vi "InitializeCamera.vi"(8 "error in (no error)":errorcluster, 11 "CameraSession in":refnum<class "CS250-CameraHardwareClass.lvclass">) -> (0 "error out":errorcluster, 3 "CameraSession out":refnum<class "CS250-CameraHardwareClass.lvclass">)   [LabVIEW 2013, in "CS250-CameraHardwareClass.lvclass"]
doc: "This VI initializes the communication with the camera and retreives the region size"
uses:
  CS250-CameraHardwareClass.lvclass
  SubVis/DLL Calls/PARAM_ID_TypDef.ctl
  CS250-CameraHardwareClass.lvclass/CS250-CameraHardwareClass.ctl
  SubVis/CamCluster.ctl
  <vilib>/vision/Image Controls.llb/IMAQ Image.ctl
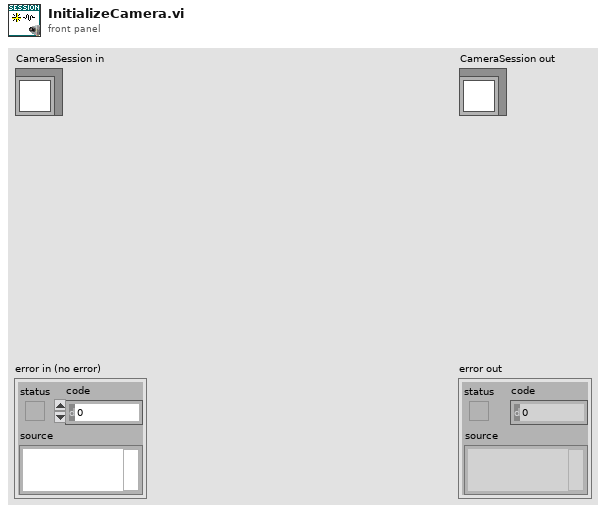
[diagram p1: front panel]
types:
  T1 = typedef "PARAM_ID_TypDef.ctl" = u32
  T2 = typedef "CamCluster.ctl" = cluster{"hcam out":i16, "TempImage":T3, "Pointer":u32, "exp_bytes out":u32, "rgn_array":cluster{"s1":u16, "s2":u16, "sbin":u16, "p1":u16, "p2":u16, "pbin":u16}, "CameraName":string}
  T3 = typedef "IMAQ Image.ctl" = refnum<image>
  T4 = cluster{"s1":u16, "s2":u16, "sbin":u16, "p1":u16, "p2":u16, "pbin":u16}
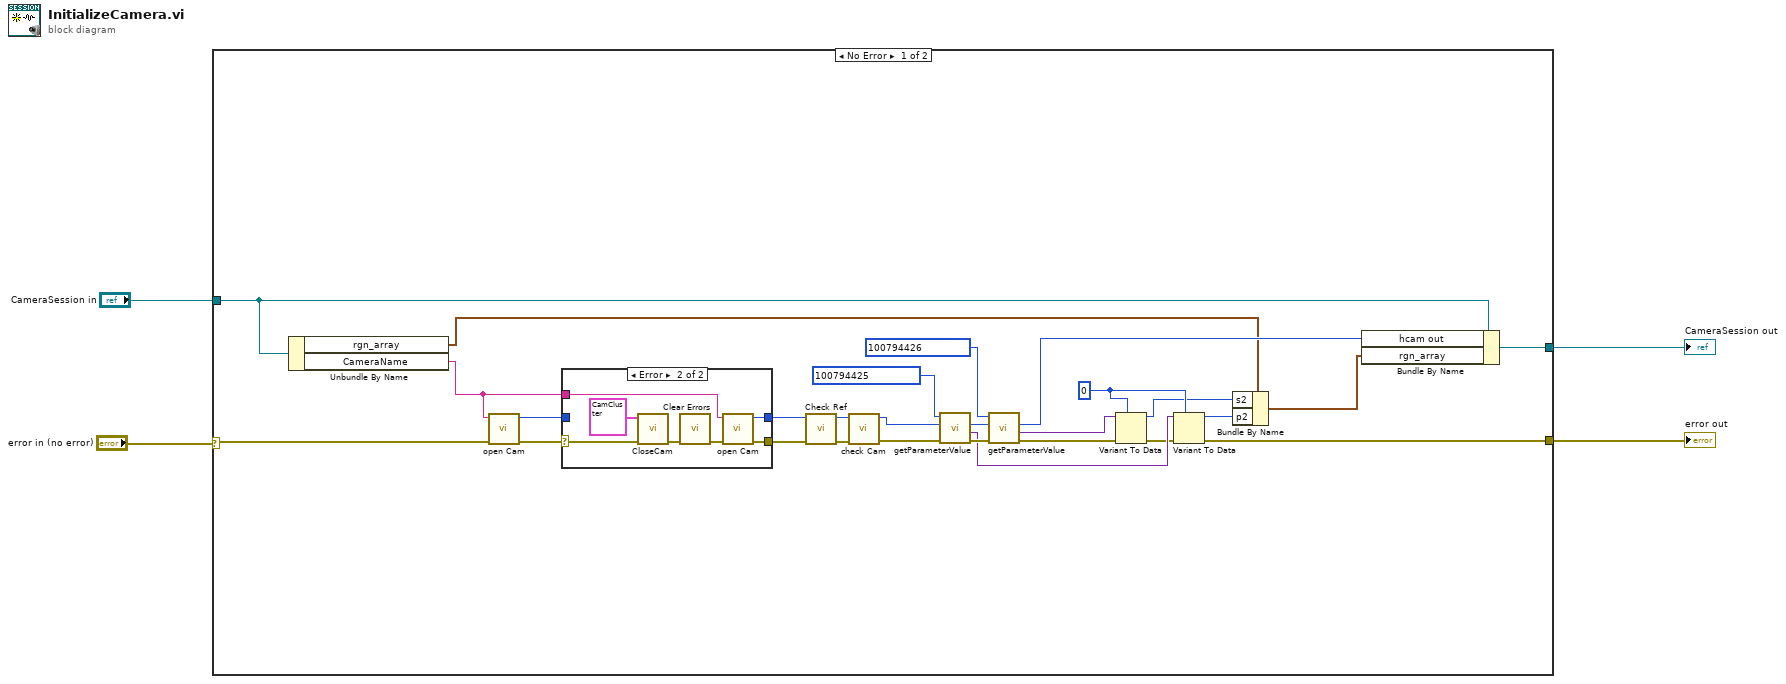
[diagram p0: block diagram]
diagram:
  n1 = case shown="No Error" "error in (no error)" {
    selector: "error in (no error)" -> [w9 w42]
    tunnel: [w8 w42] -> w3
    tunnel: [w6 w41] -> w1
    tunnel: "CameraSession in" -> [w7 w41]
    frame No Error {
      w28 = u16 0 ("s2")
      n2 = Unbundle By Name(w7) -> ("rgn_array"=w5:T4, "CameraName"=w16:string)
      n3 = call "open Cam.vi"("error in (no error)"=w9, "cam_name"=w16) -> ("error out"=w13:errorcluster, "hcam"=w15:i16)  [unwired: 8 in]
      n4 = case shown="Error" w13 {
        selector: w13 -> [w33 w34]
        tunnel: [w33 w38] -> w12
        tunnel: w16 -> [_ w37]
        tunnel: [w32 w35] -> w14
        tunnel: w15 -> [w32 _]
        frame No Error {
        }
        frame Error {
          n5 = call "CloseCam.vi"("error in (no error)"=w34, "cam cluster"=T2 {"hcam out"=0, "TempImage"="PVImage", "Pointer"=0, "exp_bytes out"=0, "rgn_array"={"s1"=0, "s2"=100, "sbin"=1, "p1"=0, "p2"=100, "pbin"=1}, "CameraName"=""} ("cam cluster out out")) -> ("error out"=w40:errorcluster)  [unwired: 9 in]
          n6 = call <vilib>:"Clear Errors.vi"("error in (no error)"=w40) -> ("error out"=w39:errorcluster)  [unwired: 6 in]
          n7 = call "open Cam.vi"("error in (no error)"=w39, "cam_name"=w37) -> ("error out"=w38:errorcluster, "hcam"=w35:i16)  [unwired: 8 in]
        }
      }
      n8 = call "Check Ref.vi"("error in (no error)"=w12, "hcam in"=w14) -> ("error out"=w11:errorcluster, "hcam out"=w10:i16)  [unwired: 8 in]
      n9 = call "check Cam.vi"("error in (no error)"=w11, "hcam out"=w10) -> ("error out"=w26:errorcluster, "hcam"=w25:i16)  [unwired: 7 in, 1 out]
      n10 = call "getParameterValue.vi"("error in (no error)"=w26, "hcam"=w25, "Param ID (Ring)"=T1 100794425) -> ("error out"=w24:errorcluster, "param_value"=w23:variant, "hcam out"=w20:i16)  [unwired: 4 in, 2 out]
      n11 = call "getParameterValue.vi"("error in (no error)"=w24, "hcam"=w20, "Param ID (Ring)"=T1 100794426) -> ("error out"=w18:errorcluster, "param_value"=w22:variant, "hcam out"=w31:i16)  [unwired: 4 in, 2 out]
      n12 = Variant To Data(error in=w18, type=w28, Variant=w22) -> (data=w27:u16, error out=w17:errorcluster)
      n13 = Variant To Data(error in=w17, type=w28, Variant=w23) -> (data=w29:u16, error out=w8:errorcluster)
      n14 = Bundle By Name(cluster=w5, "s2"=w27, "p2"=w29) -> (w30:T4)
      n15 = Bundle By Name(cluster=w7, "hcam out"=w31, "rgn_array"=w30) -> (w6:refnum<class "CS250-CameraHardwareClass.lvclass">)
    }
    frame Error {
    }
  }
  "error out" <- w3
  "CameraSession out" <- w1
